vi "Initialize Array from Array.vi"   [LabVIEW 2009]
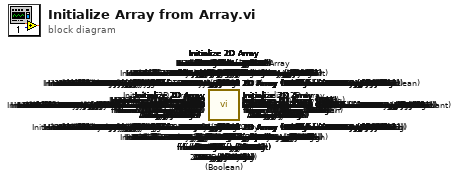
[diagram p0: block diagram]
diagram:
  n1 = call "Initialize 2D Array (Variant) from 2D Array (Variant).vi"() -> ()  [unwired: 2 in, 1 out]
  n2 = call "Initialize 2D Array (Variant) from 2D Array (U8).vi"() -> ()  [unwired: 2 in, 1 out]
  n3 = call "Initialize 2D Array (Variant) from 2D Array (U64) .vi"() -> ()  [unwired: 2 in, 1 out]
  n4 = call "Initialize 2D Array (Variant) from 2D Array (U32).vi"() -> ()  [unwired: 2 in, 1 out]
  n5 = call "Initialize 2D Array (Variant) from 2D Array (U16).vi"() -> ()  [unwired: 2 in, 1 out]
  n6 = call "Initialize 2D Array (Variant) from 2D Array (String).vi"() -> ()  [unwired: 2 in, 1 out]
  n7 = call "Initialize 2D Array (Variant) from 2D Array (SGL).vi"() -> ()  [unwired: 2 in, 1 out]
  n8 = call "Initialize 2D Array (Variant) from 2D Array (Path).vi"() -> ()  [unwired: 2 in, 1 out]
  n9 = call "Initialize 2D Array (Variant) from 2D Array (I8).vi"() -> ()  [unwired: 2 in, 1 out]
  n10 = call "Initialize 2D Array (Variant) from 2D Array (I64).vi"() -> ()  [unwired: 2 in, 1 out]
  n11 = call "Initialize 2D Array (Variant) from 2D Array (I32).vi"() -> ()  [unwired: 2 in, 1 out]
  n12 = call "Initialize 2D Array (Variant) from 2D Array (I16).vi"() -> ()  [unwired: 2 in, 1 out]
  n13 = call "Initialize 2D Array (Variant) from 2D Array (EXT).vi"() -> ()  [unwired: 2 in, 1 out]
  n14 = call "Initialize 2D Array (Variant) from 2D Array (DBL).vi"() -> ()  [unwired: 2 in, 1 out]
  n15 = call "Initialize 2D Array (Variant) from 2D Array (CXT).vi"() -> ()  [unwired: 2 in, 1 out]
  n16 = call "Initialize 2D Array (Variant) from 2D Array (CSG).vi"() -> ()  [unwired: 2 in, 1 out]
  n17 = call "Initialize 2D Array (Variant) from 2D Array (CDB).vi"() -> ()  [unwired: 2 in, 1 out]
  n18 = call "Initialize 2D Array (Variant) from 2D Array (Boolean).vi"() -> ()  [unwired: 2 in, 1 out]
  n19 = call "Initialize 2D Array (U8) from 2D Array (Variant).vi"() -> ()  [unwired: 2 in, 1 out]
  n20 = call "Initialize 2D Array (U8) from 2D Array (U8).vi"() -> ()  [unwired: 2 in, 1 out]
  n21 = call "Initialize 2D Array (U8) from 2D Array (U64) .vi"() -> ()  [unwired: 2 in, 1 out]
  n22 = call "Initialize 2D Array (U8) from 2D Array (U32).vi"() -> ()  [unwired: 2 in, 1 out]
  n23 = call "Initialize 2D Array (U8) from 2D Array (U16).vi"() -> ()  [unwired: 2 in, 1 out]
  n24 = call "Initialize 2D Array (U8) from 2D Array (String).vi"() -> ()  [unwired: 2 in, 1 out]
  n25 = call "Initialize 2D Array (U8) from 2D Array (SGL).vi"() -> ()  [unwired: 2 in, 1 out]
  n26 = call "Initialize 2D Array (U8) from 2D Array (Path).vi"() -> ()  [unwired: 2 in, 1 out]
  n27 = call "Initialize 2D Array (U8) from 2D Array (I8).vi"() -> ()  [unwired: 2 in, 1 out]
  n28 = call "Initialize 2D Array (U8) from 2D Array (I64).vi"() -> ()  [unwired: 2 in, 1 out]
  n29 = call "Initialize 2D Array (U8) from 2D Array (I32).vi"() -> ()  [unwired: 2 in, 1 out]
  n30 = call "Initialize 2D Array (U8) from 2D Array (I16).vi"() -> ()  [unwired: 2 in, 1 out]
  n31 = call "Initialize 2D Array (U8) from 2D Array (EXT).vi"() -> ()  [unwired: 2 in, 1 out]
  n32 = call "Initialize 2D Array (U8) from 2D Array (DBL).vi"() -> ()  [unwired: 2 in, 1 out]
  n33 = call "Initialize 2D Array (U8) from 2D Array (CXT).vi"() -> ()  [unwired: 2 in, 1 out]
  n34 = call "Initialize 2D Array (U8) from 2D Array (CSG).vi"() -> ()  [unwired: 2 in, 1 out]
  n35 = call "Initialize 2D Array (U8) from 2D Array (CDB).vi"() -> ()  [unwired: 2 in, 1 out]
  n36 = call "Initialize 2D Array (U8) from 2D Array (Boolean).vi"() -> ()  [unwired: 2 in, 1 out]
  n37 = call "Initialize 2D Array (U64) from 2D Array (Variant).vi"() -> ()  [unwired: 2 in, 1 out]
  n38 = call "Initialize 2D Array (U64) from 2D Array (U8).vi"() -> ()  [unwired: 2 in, 1 out]
  n39 = call "Initialize 2D Array (U64) from 2D Array (U64).vi"() -> ()  [unwired: 2 in, 1 out]
  n40 = call "Initialize 2D Array (U64) from 2D Array (U32).vi"() -> ()  [unwired: 2 in, 1 out]
  n41 = call "Initialize 2D Array (U64) from 2D Array (U16).vi"() -> ()  [unwired: 2 in, 1 out]
  n42 = call "Initialize 2D Array (U64) from 2D Array (String).vi"() -> ()  [unwired: 2 in, 1 out]
  n43 = call "Initialize 2D Array (U64) from 2D Array (SGL).vi"() -> ()  [unwired: 2 in, 1 out]
  n44 = call "Initialize 2D Array (U64) from 2D Array (Path).vi"() -> ()  [unwired: 2 in, 1 out]
  n45 = call "Initialize 2D Array (U64) from 2D Array (I8).vi"() -> ()  [unwired: 2 in, 1 out]
  n46 = call "Initialize 2D Array (U64) from 2D Array (I64).vi"() -> ()  [unwired: 2 in, 1 out]
  n47 = call "Initialize 2D Array (U64) from 2D Array (I32).vi"() -> ()  [unwired: 2 in, 1 out]
  n48 = call "Initialize 2D Array (U64) from 2D Array (I16).vi"() -> ()  [unwired: 2 in, 1 out]
  n49 = call "Initialize 2D Array (U64) from 2D Array (EXT).vi"() -> ()  [unwired: 2 in, 1 out]
  n50 = call "Initialize 2D Array (U64) from 2D Array (DBL).vi"() -> ()  [unwired: 2 in, 1 out]
  n51 = call "Initialize 2D Array (U64) from 2D Array (CXT).vi"() -> ()  [unwired: 2 in, 1 out]
  n52 = call "Initialize 2D Array (U64) from 2D Array (CSG).vi"() -> ()  [unwired: 2 in, 1 out]
  n53 = call "Initialize 2D Array (U64) from 2D Array (CDB).vi"() -> ()  [unwired: 2 in, 1 out]
  n54 = call "Initialize 2D Array (U64) from 2D Array (Boolean).vi"() -> ()  [unwired: 2 in, 1 out]
  n55 = call "Initialize 2D Array (U32) from 2D Array (Variant).vi"() -> ()  [unwired: 2 in, 1 out]
  n56 = call "Initialize 2D Array (U32) from 2D Array (U8).vi"() -> ()  [unwired: 2 in, 1 out]
  n57 = call "Initialize 2D Array (U32) from 2D Array (U64) .vi"() -> ()  [unwired: 2 in, 1 out]
  n58 = call "Initialize 2D Array (U32) from 2D Array (U32).vi"() -> ()  [unwired: 2 in, 1 out]
  n59 = call "Initialize 2D Array (U32) from 2D Array (U16).vi"() -> ()  [unwired: 2 in, 1 out]
  n60 = call "Initialize 2D Array (U32) from 2D Array (String).vi"() -> ()  [unwired: 2 in, 1 out]
  n61 = call "Initialize 2D Array (U32) from 2D Array (SGL).vi"() -> ()  [unwired: 2 in, 1 out]
  n62 = call "Initialize 2D Array (U32) from 2D Array (Path).vi"() -> ()  [unwired: 2 in, 1 out]
  n63 = call "Initialize 2D Array (U32) from 2D Array (I8).vi"() -> ()  [unwired: 2 in, 1 out]
  n64 = call "Initialize 2D Array (U32) from 2D Array (I64).vi"() -> ()  [unwired: 2 in, 1 out]
  n65 = call "Initialize 2D Array (U32) from 2D Array (I32).vi"() -> ()  [unwired: 2 in, 1 out]
  n66 = call "Initialize 2D Array (U32) from 2D Array (I16).vi"() -> ()  [unwired: 2 in, 1 out]
  n67 = call "Initialize 2D Array (U32) from 2D Array (EXT).vi"() -> ()  [unwired: 2 in, 1 out]
  n68 = call "Initialize 2D Array (U32) from 2D Array (DBL).vi"() -> ()  [unwired: 2 in, 1 out]
  n69 = call "Initialize 2D Array (U32) from 2D Array (CXT).vi"() -> ()  [unwired: 2 in, 1 out]
  n70 = call "Initialize 2D Array (U32) from 2D Array (CSG).vi"() -> ()  [unwired: 2 in, 1 out]
  n71 = call "Initialize 2D Array (U32) from 2D Array (CDB).vi"() -> ()  [unwired: 2 in, 1 out]
  n72 = call "Initialize 2D Array (U32) from 2D Array (Boolean).vi"() -> ()  [unwired: 2 in, 1 out]
  n73 = call "Initialize 2D Array (U16) from 2D Array (Variant).vi"() -> ()  [unwired: 2 in, 1 out]
  n74 = call "Initialize 2D Array (U16) from 2D Array (U8).vi"() -> ()  [unwired: 2 in, 1 out]
  n75 = call "Initialize 2D Array (U16) from 2D Array (U64) .vi"() -> ()  [unwired: 2 in, 1 out]
  n76 = call "Initialize 2D Array (U16) from 2D Array (U32).vi"() -> ()  [unwired: 2 in, 1 out]
  n77 = call "Initialize 2D Array (U16) from 2D Array (U16).vi"() -> ()  [unwired: 2 in, 1 out]
  n78 = call "Initialize 2D Array (U16) from 2D Array (String).vi"() -> ()  [unwired: 2 in, 1 out]
  n79 = call "Initialize 2D Array (U16) from 2D Array (SGL).vi"() -> ()  [unwired: 2 in, 1 out]
  n80 = call "Initialize 2D Array (U16) from 2D Array (Path).vi"() -> ()  [unwired: 2 in, 1 out]
  n81 = call "Initialize 2D Array (U16) from 2D Array (I8).vi"() -> ()  [unwired: 2 in, 1 out]
  n82 = call "Initialize 2D Array (U16) from 2D Array (I64).vi"() -> ()  [unwired: 2 in, 1 out]
  n83 = call "Initialize 2D Array (U16) from 2D Array (I32).vi"() -> ()  [unwired: 2 in, 1 out]
  n84 = call "Initialize 2D Array (U16) from 2D Array (I16).vi"() -> ()  [unwired: 2 in, 1 out]
  n85 = call "Initialize 2D Array (U16) from 2D Array (EXT).vi"() -> ()  [unwired: 2 in, 1 out]
  n86 = call "Initialize 2D Array (U16) from 2D Array (DBL).vi"() -> ()  [unwired: 2 in, 1 out]
  n87 = call "Initialize 2D Array (U16) from 2D Array (CXT).vi"() -> ()  [unwired: 2 in, 1 out]
  n88 = call "Initialize 2D Array (U16) from 2D Array (CSG).vi"() -> ()  [unwired: 2 in, 1 out]
  n89 = call "Initialize 2D Array (U16) from 2D Array (CDB).vi"() -> ()  [unwired: 2 in, 1 out]
  n90 = call "Initialize 2D Array (U16) from 2D Array (Boolean).vi"() -> ()  [unwired: 2 in, 1 out]
  n91 = call "Initialize 2D Array (String) from 2D Array (Variant).vi"() -> ()  [unwired: 2 in, 1 out]
  n92 = call "Initialize 2D Array (String) from 2D Array (U8).vi"() -> ()  [unwired: 2 in, 1 out]
  n93 = call "Initialize 2D Array (String) from 2D Array (U64) .vi"() -> ()  [unwired: 2 in, 1 out]
  n94 = call "Initialize 2D Array (String) from 2D Array (U32).vi"() -> ()  [unwired: 2 in, 1 out]
  n95 = call "Initialize 2D Array (String) from 2D Array (U16).vi"() -> ()  [unwired: 2 in, 1 out]
  n96 = call "Initialize 2D Array (String) from 2D Array (String).vi"() -> ()  [unwired: 2 in, 1 out]
  n97 = call "Initialize 2D Array (String) from 2D Array (SGL).vi"() -> ()  [unwired: 2 in, 1 out]
  n98 = call "Initialize 2D Array (String) from 2D Array (Path).vi"() -> ()  [unwired: 2 in, 1 out]
  n99 = call "Initialize 2D Array (String) from 2D Array (I8).vi"() -> ()  [unwired: 2 in, 1 out]
  n100 = call "Initialize 2D Array (String) from 2D Array (I64).vi"() -> ()  [unwired: 2 in, 1 out]
  n101 = call "Initialize 2D Array (String) from 2D Array (I32).vi"() -> ()  [unwired: 2 in, 1 out]
  n102 = call "Initialize 2D Array (String) from 2D Array (I16).vi"() -> ()  [unwired: 2 in, 1 out]
  n103 = call "Initialize 2D Array (String) from 2D Array (EXT).vi"() -> ()  [unwired: 2 in, 1 out]
  n104 = call "Initialize 2D Array (String) from 2D Array (DBL).vi"() -> ()  [unwired: 2 in, 1 out]
  n105 = call "Initialize 2D Array (String) from 2D Array (CXT).vi"() -> ()  [unwired: 2 in, 1 out]
  n106 = call "Initialize 2D Array (String) from 2D Array (CSG).vi"() -> ()  [unwired: 2 in, 1 out]
  n107 = call "Initialize 2D Array (String) from 2D Array (CDB).vi"() -> ()  [unwired: 2 in, 1 out]
  n108 = call "Initialize 2D Array (String) from 2D Array (Boolean).vi"() -> ()  [unwired: 2 in, 1 out]
  n109 = call "Initialize 2D Array (SGL) from 2D Array (Variant).vi"() -> ()  [unwired: 2 in, 1 out]
  n110 = call "Initialize 2D Array (SGL) from 2D Array (U8).vi"() -> ()  [unwired: 2 in, 1 out]
  n111 = call "Initialize 2D Array (SGL) from 2D Array (U64) .vi"() -> ()  [unwired: 2 in, 1 out]
  n112 = call "Initialize 2D Array (SGL) from 2D Array (U32).vi"() -> ()  [unwired: 2 in, 1 out]
  n113 = call "Initialize 2D Array (SGL) from 2D Array (U16).vi"() -> ()  [unwired: 2 in, 1 out]
  n114 = call "Initialize 2D Array (SGL) from 2D Array (String).vi"() -> ()  [unwired: 2 in, 1 out]
  n115 = call "Initialize 2D Array (SGL) from 2D Array (SGL).vi"() -> ()  [unwired: 2 in, 1 out]
  n116 = call "Initialize 2D Array (SGL) from 2D Array (Path).vi"() -> ()  [unwired: 2 in, 1 out]
  n117 = call "Initialize 2D Array (SGL) from 2D Array (I8).vi"() -> ()  [unwired: 2 in, 1 out]
  n118 = call "Initialize 2D Array (SGL) from 2D Array (I64).vi"() -> ()  [unwired: 2 in, 1 out]
  n119 = call "Initialize 2D Array (SGL) from 2D Array (I32).vi"() -> ()  [unwired: 2 in, 1 out]
  n120 = call "Initialize 2D Array (SGL) from 2D Array (I16).vi"() -> ()  [unwired: 2 in, 1 out]
  n121 = call "Initialize 2D Array (SGL) from 2D Array (EXT).vi"() -> ()  [unwired: 2 in, 1 out]
  n122 = call "Initialize 2D Array (SGL) from 2D Array (DBL).vi"() -> ()  [unwired: 2 in, 1 out]
  n123 = call "Initialize 2D Array (SGL) from 2D Array (CXT).vi"() -> ()  [unwired: 2 in, 1 out]
  n124 = call "Initialize 2D Array (SGL) from 2D Array (CSG).vi"() -> ()  [unwired: 2 in, 1 out]
  n125 = call "Initialize 2D Array (SGL) from 2D Array (CDB).vi"() -> ()  [unwired: 2 in, 1 out]
  n126 = call "Initialize 2D Array (SGL) from 2D Array (Boolean).vi"() -> ()  [unwired: 2 in, 1 out]
  n127 = call "Initialize 2D Array (Path) from 2D Array (Variant).vi"() -> ()  [unwired: 2 in, 1 out]
  n128 = call "Initialize 2D Array (Path) from 2D Array (U8).vi"() -> ()  [unwired: 2 in, 1 out]
  n129 = call "Initialize 2D Array (Path) from 2D Array (U64) .vi"() -> ()  [unwired: 2 in, 1 out]
  n130 = call "Initialize 2D Array (Path) from 2D Array (U32).vi"() -> ()  [unwired: 2 in, 1 out]
  n131 = call "Initialize 2D Array (Path) from 2D Array (U16).vi"() -> ()  [unwired: 2 in, 1 out]
  n132 = call "Initialize 2D Array (Path) from 2D Array (String).vi"() -> ()  [unwired: 2 in, 1 out]
  n133 = call "Initialize 2D Array (Path) from 2D Array (SGL).vi"() -> ()  [unwired: 2 in, 1 out]
  n134 = call "Initialize 2D Array (Path) from 2D Array (Path).vi"() -> ()  [unwired: 2 in, 1 out]
  n135 = call "Initialize 2D Array (Path) from 2D Array (I8).vi"() -> ()  [unwired: 2 in, 1 out]
  n136 = call "Initialize 2D Array (Path) from 2D Array (I64).vi"() -> ()  [unwired: 2 in, 1 out]
  n137 = call "Initialize 2D Array (Path) from 2D Array (I32).vi"() -> ()  [unwired: 2 in, 1 out]
  n138 = call "Initialize 2D Array (Path) from 2D Array (I16).vi"() -> ()  [unwired: 2 in, 1 out]
  n139 = call "Initialize 2D Array (Path) from 2D Array (EXT).vi"() -> ()  [unwired: 2 in, 1 out]
  n140 = call "Initialize 2D Array (Path) from 2D Array (DBL).vi"() -> ()  [unwired: 2 in, 1 out]
  n141 = call "Initialize 2D Array (Path) from 2D Array (CXT).vi"() -> ()  [unwired: 2 in, 1 out]
  n142 = call "Initialize 2D Array (Path) from 2D Array (CSG).vi"() -> ()  [unwired: 2 in, 1 out]
  n143 = call "Initialize 2D Array (Path) from 2D Array (CDB).vi"() -> ()  [unwired: 2 in, 1 out]
  n144 = call "Initialize 2D Array (Path) from 2D Array (Boolean).vi"() -> ()  [unwired: 2 in, 1 out]
  n145 = call "Initialize 2D Array (I8) from 2D Array (Variant).vi"() -> ()  [unwired: 2 in, 1 out]
  n146 = call "Initialize 2D Array (I8) from 2D Array (U8).vi"() -> ()  [unwired: 2 in, 1 out]
  n147 = call "Initialize 2D Array (I8) from 2D Array (U64) .vi"() -> ()  [unwired: 2 in, 1 out]
  n148 = call "Initialize 2D Array (I8) from 2D Array (U32).vi"() -> ()  [unwired: 2 in, 1 out]
  n149 = call "Initialize 2D Array (I8) from 2D Array (U16).vi"() -> ()  [unwired: 2 in, 1 out]
  n150 = call "Initialize 2D Array (I8) from 2D Array (String).vi"() -> ()  [unwired: 2 in, 1 out]
  n151 = call "Initialize 2D Array (I8) from 2D Array (SGL).vi"() -> ()  [unwired: 2 in, 1 out]
  n152 = call "Initialize 2D Array (I8) from 2D Array (Path).vi"() -> ()  [unwired: 2 in, 1 out]
  n153 = call "Initialize 2D Array (I8) from 2D Array (I8).vi"() -> ()  [unwired: 2 in, 1 out]
  n154 = call "Initialize 2D Array (I8) from 2D Array (I64).vi"() -> ()  [unwired: 2 in, 1 out]
  n155 = call "Initialize 2D Array (I8) from 2D Array (I32).vi"() -> ()  [unwired: 2 in, 1 out]
  n156 = call "Initialize 2D Array (I8) from 2D Array (I16).vi"() -> ()  [unwired: 2 in, 1 out]
  n157 = call "Initialize 2D Array (I8) from 2D Array (EXT).vi"() -> ()  [unwired: 2 in, 1 out]
  n158 = call "Initialize 2D Array (I8) from 2D Array (DBL).vi"() -> ()  [unwired: 2 in, 1 out]
  n159 = call "Initialize 2D Array (I8) from 2D Array (CXT).vi"() -> ()  [unwired: 2 in, 1 out]
  n160 = call "Initialize 2D Array (I8) from 2D Array (CSG).vi"() -> ()  [unwired: 2 in, 1 out]
  n161 = call "Initialize 2D Array (I8) from 2D Array (CDB).vi"() -> ()  [unwired: 2 in, 1 out]
  n162 = call "Initialize 2D Array (I8) from 2D Array (Boolean).vi"() -> ()  [unwired: 2 in, 1 out]
  n163 = call "Initialize 2D Array (I64) from 2D Array (Variant).vi"() -> ()  [unwired: 2 in, 1 out]
  n164 = call "Initialize 2D Array (I64) from 2D Array (U8).vi"() -> ()  [unwired: 2 in, 1 out]
  n165 = call "Initialize 2D Array (I64) from 2D Array (U64).vi"() -> ()  [unwired: 2 in, 1 out]
  n166 = call "Initialize 2D Array (I64) from 2D Array (U32).vi"() -> ()  [unwired: 2 in, 1 out]
  n167 = call "Initialize 2D Array (I64) from 2D Array (U16).vi"() -> ()  [unwired: 2 in, 1 out]
  n168 = call "Initialize 2D Array (I64) from 2D Array (String).vi"() -> ()  [unwired: 2 in, 1 out]
  n169 = call "Initialize 2D Array (I64) from 2D Array (SGL).vi"() -> ()  [unwired: 2 in, 1 out]
  n170 = call "Initialize 2D Array (I64) from 2D Array (Path).vi"() -> ()  [unwired: 2 in, 1 out]
  n171 = call "Initialize 2D Array (I64) from 2D Array (I8).vi"() -> ()  [unwired: 2 in, 1 out]
  n172 = call "Initialize 2D Array (I64) from 2D Array (I64).vi"() -> ()  [unwired: 2 in, 1 out]
  n173 = call "Initialize 2D Array (I64) from 2D Array (I32).vi"() -> ()  [unwired: 2 in, 1 out]
  n174 = call "Initialize 2D Array (I64) from 2D Array (I16).vi"() -> ()  [unwired: 2 in, 1 out]
  n175 = call "Initialize 2D Array (I64) from 2D Array (EXT).vi"() -> ()  [unwired: 2 in, 1 out]
  n176 = call "Initialize 2D Array (I64) from 2D Array (DBL).vi"() -> ()  [unwired: 2 in, 1 out]
  n177 = call "Initialize 2D Array (I64) from 2D Array (CXT).vi"() -> ()  [unwired: 2 in, 1 out]
  n178 = call "Initialize 2D Array (I64) from 2D Array (CSG).vi"() -> ()  [unwired: 2 in, 1 out]
  n179 = call "Initialize 2D Array (I64) from 2D Array (CDB).vi"() -> ()  [unwired: 2 in, 1 out]
  n180 = call "Initialize 2D Array (I64) from 2D Array (Boolean).vi"() -> ()  [unwired: 2 in, 1 out]
  n181 = call "Initialize 2D Array (I32) from 2D Array (Variant).vi"() -> ()  [unwired: 2 in, 1 out]
  n182 = call "Initialize 2D Array (I32) from 2D Array (U8).vi"() -> ()  [unwired: 2 in, 1 out]
  n183 = call "Initialize 2D Array (I32) from 2D Array (U64) .vi"() -> ()  [unwired: 2 in, 1 out]
  n184 = call "Initialize 2D Array (I32) from 2D Array (U32).vi"() -> ()  [unwired: 2 in, 1 out]
  n185 = call "Initialize 2D Array (I32) from 2D Array (U16).vi"() -> ()  [unwired: 2 in, 1 out]
  n186 = call "Initialize 2D Array (I32) from 2D Array (String).vi"() -> ()  [unwired: 2 in, 1 out]
  n187 = call "Initialize 2D Array (I32) from 2D Array (SGL).vi"() -> ()  [unwired: 2 in, 1 out]
  n188 = call "Initialize 2D Array (I32) from 2D Array (Path).vi"() -> ()  [unwired: 2 in, 1 out]
  n189 = call "Initialize 2D Array (I32) from 2D Array (I8).vi"() -> ()  [unwired: 2 in, 1 out]
  n190 = call "Initialize 2D Array (I32) from 2D Array (I64).vi"() -> ()  [unwired: 2 in, 1 out]
  n191 = call "Initialize 2D Array (I32) from 2D Array (I32).vi"() -> ()  [unwired: 2 in, 1 out]
  n192 = call "Initialize 2D Array (I32) from 2D Array (I16).vi"() -> ()  [unwired: 2 in, 1 out]
  n193 = call "Initialize 2D Array (I32) from 2D Array (EXT).vi"() -> ()  [unwired: 2 in, 1 out]
  n194 = call "Initialize 2D Array (I32) from 2D Array (DBL).vi"() -> ()  [unwired: 2 in, 1 out]
  n195 = call "Initialize 2D Array (I32) from 2D Array (CXT).vi"() -> ()  [unwired: 2 in, 1 out]
  n196 = call "Initialize 2D Array (I32) from 2D Array (CSG).vi"() -> ()  [unwired: 2 in, 1 out]
  n197 = call "Initialize 2D Array (I32) from 2D Array (CDB).vi"() -> ()  [unwired: 2 in, 1 out]
  n198 = call "Initialize 2D Array (I32) from 2D Array (Boolean).vi"() -> ()  [unwired: 2 in, 1 out]
  n199 = call "Initialize 2D Array (I16) from 2D Array (Variant).vi"() -> ()  [unwired: 2 in, 1 out]
  n200 = call "Initialize 2D Array (I16) from 2D Array (U8).vi"() -> ()  [unwired: 2 in, 1 out]
  n201 = call "Initialize 2D Array (I16) from 2D Array (U64) .vi"() -> ()  [unwired: 2 in, 1 out]
  n202 = call "Initialize 2D Array (I16) from 2D Array (U32).vi"() -> ()  [unwired: 2 in, 1 out]
  n203 = call "Initialize 2D Array (I16) from 2D Array (U16).vi"() -> ()  [unwired: 2 in, 1 out]
  n204 = call "Initialize 2D Array (I16) from 2D Array (String).vi"() -> ()  [unwired: 2 in, 1 out]
  n205 = call "Initialize 2D Array (I16) from 2D Array (SGL).vi"() -> ()  [unwired: 2 in, 1 out]
  n206 = call "Initialize 2D Array (I16) from 2D Array (Path).vi"() -> ()  [unwired: 2 in, 1 out]
  n207 = call "Initialize 2D Array (I16) from 2D Array (I8).vi"() -> ()  [unwired: 2 in, 1 out]
  n208 = call "Initialize 2D Array (I16) from 2D Array (I64).vi"() -> ()  [unwired: 2 in, 1 out]
  n209 = call "Initialize 2D Array (I16) from 2D Array (I32).vi"() -> ()  [unwired: 2 in, 1 out]
  n210 = call "Initialize 2D Array (I16) from 2D Array (I16).vi"() -> ()  [unwired: 2 in, 1 out]
  n211 = call "Initialize 2D Array (I16) from 2D Array (EXT).vi"() -> ()  [unwired: 2 in, 1 out]
  n212 = call "Initialize 2D Array (I16) from 2D Array (DBL).vi"() -> ()  [unwired: 2 in, 1 out]
  n213 = call "Initialize 2D Array (I16) from 2D Array (CXT).vi"() -> ()  [unwired: 2 in, 1 out]
  n214 = call "Initialize 2D Array (I16) from 2D Array (CSG).vi"() -> ()  [unwired: 2 in, 1 out]
  n215 = call "Initialize 2D Array (I16) from 2D Array (CDB).vi"() -> ()  [unwired: 2 in, 1 out]
  n216 = call "Initialize 2D Array (I16) from 2D Array (Boolean).vi"() -> ()  [unwired: 2 in, 1 out]
  n217 = call "Initialize 2D Array (EXT) from 2D Array (Variant).vi"() -> ()  [unwired: 2 in, 1 out]
  n218 = call "Initialize 2D Array (EXT) from 2D Array (U8).vi"() -> ()  [unwired: 2 in, 1 out]
  n219 = call "Initialize 2D Array (EXT) from 2D Array (U64) .vi"() -> ()  [unwired: 2 in, 1 out]
  n220 = call "Initialize 2D Array (EXT) from 2D Array (U32).vi"() -> ()  [unwired: 2 in, 1 out]
  n221 = call "Initialize 2D Array (EXT) from 2D Array (U16).vi"() -> ()  [unwired: 2 in, 1 out]
  n222 = call "Initialize 2D Array (EXT) from 2D Array (String).vi"() -> ()  [unwired: 2 in, 1 out]
  n223 = call "Initialize 2D Array (EXT) from 2D Array (SGL).vi"() -> ()  [unwired: 2 in, 1 out]
  n224 = call "Initialize 2D Array (EXT) from 2D Array (Path).vi"() -> ()  [unwired: 2 in, 1 out]
  n225 = call "Initialize 2D Array (EXT) from 2D Array (I8).vi"() -> ()  [unwired: 2 in, 1 out]
  n226 = call "Initialize 2D Array (EXT) from 2D Array (I64).vi"() -> ()  [unwired: 2 in, 1 out]
  n227 = call "Initialize 2D Array (EXT) from 2D Array (I32).vi"() -> ()  [unwired: 2 in, 1 out]
  n228 = call "Initialize 2D Array (EXT) from 2D Array (I16).vi"() -> ()  [unwired: 2 in, 1 out]
  n229 = call "Initialize 2D Array (EXT) from 2D Array (EXT).vi"() -> ()  [unwired: 2 in, 1 out]
  n230 = call "Initialize 2D Array (EXT) from 2D Array (DBL).vi"() -> ()  [unwired: 2 in, 1 out]
  n231 = call "Initialize 2D Array (EXT) from 2D Array (CXT).vi"() -> ()  [unwired: 2 in, 1 out]
  n232 = call "Initialize 2D Array (EXT) from 2D Array (CSG).vi"() -> ()  [unwired: 2 in, 1 out]
  n233 = call "Initialize 2D Array (EXT) from 2D Array (CDB).vi"() -> ()  [unwired: 2 in, 1 out]
  n234 = call "Initialize 2D Array (EXT) from 2D Array (Boolean).vi"() -> ()  [unwired: 2 in, 1 out]
  n235 = call "Initialize 2D Array (DBL) from 2D Array (Variant).vi"() -> ()  [unwired: 2 in, 1 out]
  n236 = call "Initialize 2D Array (DBL) from 2D Array (U8).vi"() -> ()  [unwired: 2 in, 1 out]
  n237 = call "Initialize 2D Array (DBL) from 2D Array (U64) .vi"() -> ()  [unwired: 2 in, 1 out]
  n238 = call "Initialize 2D Array (DBL) from 2D Array (U32).vi"() -> ()  [unwired: 2 in, 1 out]
  n239 = call "Initialize 2D Array (DBL) from 2D Array (U16).vi"() -> ()  [unwired: 2 in, 1 out]
  n240 = call "Initialize 2D Array (DBL) from 2D Array (String).vi"() -> ()  [unwired: 2 in, 1 out]
  n241 = call "Initialize 2D Array (DBL) from 2D Array (SGL).vi"() -> ()  [unwired: 2 in, 1 out]
  n242 = call "Initialize 2D Array (DBL) from 2D Array (Path).vi"() -> ()  [unwired: 2 in, 1 out]
  n243 = call "Initialize 2D Array (DBL) from 2D Array (I8).vi"() -> ()  [unwired: 2 in, 1 out]
  n244 = call "Initialize 2D Array (DBL) from 2D Array (I64).vi"() -> ()  [unwired: 2 in, 1 out]
  n245 = call "Initialize 2D Array (DBL) from 2D Array (I32).vi"() -> ()  [unwired: 2 in, 1 out]
  n246 = call "Initialize 2D Array (DBL) from 2D Array (I16).vi"() -> ()  [unwired: 2 in, 1 out]
  n247 = call "Initialize 2D Array (DBL) from 2D Array (EXT).vi"() -> ()  [unwired: 2 in, 1 out]
  n248 = call "Initialize 2D Array (DBL) from 2D Array (DBL).vi"() -> ()  [unwired: 2 in, 1 out]
  n249 = call "Initialize 2D Array (DBL) from 2D Array (CXT).vi"() -> ()  [unwired: 2 in, 1 out]
  n250 = call "Initialize 2D Array (DBL) from 2D Array (CSG).vi"() -> ()  [unwired: 2 in, 1 out]
  n251 = call "Initialize 2D Array (DBL) from 2D Array (CDB).vi"() -> ()  [unwired: 2 in, 1 out]
  n252 = call "Initialize 2D Array (DBL) from 2D Array (Boolean).vi"() -> ()  [unwired: 2 in, 1 out]
  n253 = call "Initialize 2D Array (CXT) from 2D Array (Variant).vi"() -> ()  [unwired: 2 in, 1 out]
  n254 = call "Initialize 2D Array (CXT) from 2D Array (U8).vi"() -> ()  [unwired: 2 in, 1 out]
  n255 = call "Initialize 2D Array (CXT) from 2D Array (U64) .vi"() -> ()  [unwired: 2 in, 1 out]
  n256 = call "Initialize 2D Array (CXT) from 2D Array (U32).vi"() -> ()  [unwired: 2 in, 1 out]
  n257 = call "Initialize 2D Array (CXT) from 2D Array (U16).vi"() -> ()  [unwired: 2 in, 1 out]
  n258 = call "Initialize 2D Array (CXT) from 2D Array (String).vi"() -> ()  [unwired: 2 in, 1 out]
  n259 = call "Initialize 2D Array (CXT) from 2D Array (SGL).vi"() -> ()  [unwired: 2 in, 1 out]
  n260 = call "Initialize 2D Array (CXT) from 2D Array (Path).vi"() -> ()  [unwired: 2 in, 1 out]
  n261 = call "Initialize 2D Array (CXT) from 2D Array (I8).vi"() -> ()  [unwired: 2 in, 1 out]
  n262 = call "Initialize 2D Array (CXT) from 2D Array (I64).vi"() -> ()  [unwired: 2 in, 1 out]
  n263 = call "Initialize 2D Array (CXT) from 2D Array (I32).vi"() -> ()  [unwired: 2 in, 1 out]
  n264 = call "Initialize 2D Array (CXT) from 2D Array (I16).vi"() -> ()  [unwired: 2 in, 1 out]
  n265 = call "Initialize 2D Array (CXT) from 2D Array (EXT).vi"() -> ()  [unwired: 2 in, 1 out]
  n266 = call "Initialize 2D Array (CXT) from 2D Array (DBL).vi"() -> ()  [unwired: 2 in, 1 out]
  n267 = call "Initialize 2D Array (CXT) from 2D Array (CXT).vi"() -> ()  [unwired: 2 in, 1 out]
  n268 = call "Initialize 2D Array (CXT) from 2D Array (CSG).vi"() -> ()  [unwired: 2 in, 1 out]
  n269 = call "Initialize 2D Array (CXT) from 2D Array (CDB).vi"() -> ()  [unwired: 2 in, 1 out]
  n270 = call "Initialize 2D Array (CXT) from 2D Array (Boolean).vi"() -> ()  [unwired: 2 in, 1 out]
  n271 = call "Initialize 2D Array (CSG) from 2D Array (Variant).vi"() -> ()  [unwired: 2 in, 1 out]
  n272 = call "Initialize 2D Array (CSG) from 2D Array (U8).vi"() -> ()  [unwired: 2 in, 1 out]
  n273 = call "Initialize 2D Array (CSG) from 2D Array (U64) .vi"() -> ()  [unwired: 2 in, 1 out]
  n274 = call "Initialize 2D Array (CSG) from 2D Array (U32).vi"() -> ()  [unwired: 2 in, 1 out]
  n275 = call "Initialize 2D Array (CSG) from 2D Array (U16).vi"() -> ()  [unwired: 2 in, 1 out]
  n276 = call "Initialize 2D Array (CSG) from 2D Array (String).vi"() -> ()  [unwired: 2 in, 1 out]
  n277 = call "Initialize 2D Array (CSG) from 2D Array (SGL).vi"() -> ()  [unwired: 2 in, 1 out]
  n278 = call "Initialize 2D Array (CSG) from 2D Array (Path).vi"() -> ()  [unwired: 2 in, 1 out]
  n279 = call "Initialize 2D Array (CSG) from 2D Array (I8).vi"() -> ()  [unwired: 2 in, 1 out]
  n280 = call "Initialize 2D Array (CSG) from 2D Array (I64).vi"() -> ()  [unwired: 2 in, 1 out]
  n281 = call "Initialize 2D Array (CSG) from 2D Array (I32).vi"() -> ()  [unwired: 2 in, 1 out]
  n282 = call "Initialize 2D Array (CSG) from 2D Array (I16).vi"() -> ()  [unwired: 2 in, 1 out]
  n283 = call "Initialize 2D Array (CSG) from 2D Array (EXT).vi"() -> ()  [unwired: 2 in, 1 out]
  n284 = call "Initialize 2D Array (CSG) from 2D Array (DBL).vi"() -> ()  [unwired: 2 in, 1 out]
  n285 = call "Initialize 2D Array (CSG) from 2D Array (CXT).vi"() -> ()  [unwired: 2 in, 1 out]
  n286 = call "Initialize 2D Array (CSG) from 2D Array (CSG).vi"() -> ()  [unwired: 2 in, 1 out]
  n287 = call "Initialize 2D Array (CSG) from 2D Array (CDB).vi"() -> ()  [unwired: 2 in, 1 out]
  n288 = call "Initialize 2D Array (CSG) from 2D Array (Boolean).vi"() -> ()  [unwired: 2 in, 1 out]
  n289 = call "Initialize 2D Array (CDB) from 2D Array (Variant).vi"() -> ()  [unwired: 2 in, 1 out]
  n290 = call "Initialize 2D Array (CDB) from 2D Array (U8).vi"() -> ()  [unwired: 2 in, 1 out]
  n291 = call "Initialize 2D Array (CDB) from 2D Array (U64) .vi"() -> ()  [unwired: 2 in, 1 out]
  n292 = call "Initialize 2D Array (CDB) from 2D Array (U32).vi"() -> ()  [unwired: 2 in, 1 out]
  n293 = call "Initialize 2D Array (CDB) from 2D Array (U16).vi"() -> ()  [unwired: 2 in, 1 out]
  n294 = call "Initialize 2D Array (CDB) from 2D Array (String).vi"() -> ()  [unwired: 2 in, 1 out]
  n295 = call "Initialize 2D Array (CDB) from 2D Array (SGL).vi"() -> ()  [unwired: 2 in, 1 out]
  n296 = call "Initialize 2D Array (CDB) from 2D Array (Path).vi"() -> ()  [unwired: 2 in, 1 out]
  n297 = call "Initialize 2D Array (CDB) from 2D Array (I8).vi"() -> ()  [unwired: 2 in, 1 out]
  n298 = call "Initialize 2D Array (CDB) from 2D Array (I64).vi"() -> ()  [unwired: 2 in, 1 out]
  n299 = call "Initialize 2D Array (CDB) from 2D Array (I32).vi"() -> ()  [unwired: 2 in, 1 out]
  n300 = call "Initialize 2D Array (CDB) from 2D Array (I16).vi"() -> ()  [unwired: 2 in, 1 out]
  n301 = call "Initialize 2D Array (CDB) from 2D Array (EXT).vi"() -> ()  [unwired: 2 in, 1 out]
  n302 = call "Initialize 2D Array (CDB) from 2D Array (DBL).vi"() -> ()  [unwired: 2 in, 1 out]
  n303 = call "Initialize 2D Array (CDB) from 2D Array (CXT).vi"() -> ()  [unwired: 2 in, 1 out]
  n304 = call "Initialize 2D Array (CDB) from 2D Array (CSG).vi"() -> ()  [unwired: 2 in, 1 out]
  n305 = call "Initialize 2D Array (CDB) from 2D Array (CDB).vi"() -> ()  [unwired: 2 in, 1 out]
  n306 = call "Initialize 2D Array (CDB) from 2D Array (Boolean).vi"() -> ()  [unwired: 2 in, 1 out]
  n307 = call "Initialize 2D Array (Boolean) from 2D Array (Variant).vi"() -> ()  [unwired: 2 in, 1 out]
  n308 = call "Initialize 2D Array (Boolean) from 2D Array (U8).vi"() -> ()  [unwired: 2 in, 1 out]
  n309 = call "Initialize 2D Array (Boolean) from 2D Array (U64) .vi"() -> ()  [unwired: 2 in, 1 out]
  n310 = call "Initialize 2D Array (Boolean) from 2D Array (U32).vi"() -> ()  [unwired: 2 in, 1 out]
  n311 = call "Initialize 2D Array (Boolean) from 2D Array (U16).vi"() -> ()  [unwired: 2 in, 1 out]
  n312 = call "Initialize 2D Array (Boolean) from 2D Array (String).vi"() -> ()  [unwired: 2 in, 1 out]
  n313 = call "Initialize 2D Array (Boolean) from 2D Array (SGL).vi"() -> ()  [unwired: 2 in, 1 out]
  n314 = call "Initialize 2D Array (Boolean) from 2D Array (Path).vi"() -> ()  [unwired: 2 in, 1 out]
  n315 = call "Initialize 2D Array (Boolean) from 2D Array (I8).vi"() -> ()  [unwired: 2 in, 1 out]
  n316 = call "Initialize 2D Array (Boolean) from 2D Array (I64).vi"() -> ()  [unwired: 2 in, 1 out]
  n317 = call "Initialize 2D Array (Boolean) from 2D Array (I32).vi"() -> ()  [unwired: 2 in, 1 out]
  n318 = call "Initialize 2D Array (Boolean) from 2D Array (I16).vi"() -> ()  [unwired: 2 in, 1 out]
  n319 = call "Initialize 2D Array (Boolean) from 2D Array (EXT).vi"() -> ()  [unwired: 2 in, 1 out]
  n320 = call "Initialize 2D Array (Boolean) from 2D Array (DBL).vi"() -> ()  [unwired: 2 in, 1 out]
  n321 = call "Initialize 2D Array (Boolean) from 2D Array (CXT).vi"() -> ()  [unwired: 2 in, 1 out]
  n322 = call "Initialize 2D Array (Boolean) from 2D Array (CSG).vi"() -> ()  [unwired: 2 in, 1 out]
  n323 = call "Initialize 2D Array (Boolean) from 2D Array (CDB).vi"() -> ()  [unwired: 2 in, 1 out]
  n324 = call "Initialize 2D Array (Boolean) from 2D Array (Boolean).vi"() -> ()  [unwired: 2 in, 1 out]
  n325 = call "Initialize 1D Array (Variant) from 1D Array (Variant).vi"() -> ()  [unwired: 2 in, 1 out]
  n326 = call "Initialize 1D Array (Variant) from 1D Array (U8).vi"() -> ()  [unwired: 2 in, 1 out]
  n327 = call "Initialize 1D Array (Variant) from 1D Array (U64).vi"() -> ()  [unwired: 2 in, 1 out]
  n328 = call "Initialize 1D Array (Variant) from 1D Array (U32).vi"() -> ()  [unwired: 2 in, 1 out]
  n329 = call "Initialize 1D Array (Variant) from 1D Array (U16).vi"() -> ()  [unwired: 2 in, 1 out]
  n330 = call "Initialize 1D Array (Variant) from 1D Array (String).vi"() -> ()  [unwired: 2 in, 1 out]
  n331 = call "Initialize 1D Array (Variant) from 1D Array (SGL).vi"() -> ()  [unwired: 2 in, 1 out]
  n332 = call "Initialize 1D Array (Variant) from 1D Array (Path).vi"() -> ()  [unwired: 2 in, 1 out]
  n333 = call "Initialize 1D Array (Variant) from 1D Array (I8).vi"() -> ()  [unwired: 2 in, 1 out]
  n334 = call "Initialize 1D Array (Variant) from 1D Array (I64).vi"() -> ()  [unwired: 2 in, 1 out]
  n335 = call "Initialize 1D Array (Variant) from 1D Array (I32).vi"() -> ()  [unwired: 2 in, 1 out]
  n336 = call "Initialize 1D Array (Variant) from 1D Array (I16).vi"() -> ()  [unwired: 2 in, 1 out]
  n337 = call "Initialize 1D Array (Variant) from 1D Array (EXT).vi"() -> ()  [unwired: 2 in, 1 out]
  n338 = call "Initialize 1D Array (Variant) from 1D Array (DBL).vi"() -> ()  [unwired: 2 in, 1 out]
  n339 = call "Initialize 1D Array (Variant) from 1D Array (CXT).vi"() -> ()  [unwired: 2 in, 1 out]
  n340 = call "Initialize 1D Array (Variant) from 1D Array (CSG).vi"() -> ()  [unwired: 2 in, 1 out]
  n341 = call "Initialize 1D Array (Variant) from 1D Array (CDB).vi"() -> ()  [unwired: 2 in, 1 out]
  n342 = call "Initialize 1D Array (Variant) from 1D Array (Boolean).vi"() -> ()  [unwired: 2 in, 1 out]
  n343 = call "Initialize 1D Array (U8) from 1D Array (Variant).vi"() -> ()  [unwired: 2 in, 1 out]
  n344 = call "Initialize 1D Array (U8) from 1D Array (U8).vi"() -> ()  [unwired: 2 in, 1 out]
  n345 = call "Initialize 1D Array (U8) from 1D Array (U64).vi"() -> ()  [unwired: 2 in, 1 out]
  n346 = call "Initialize 1D Array (U8) from 1D Array (U32).vi"() -> ()  [unwired: 2 in, 1 out]
  n347 = call "Initialize 1D Array (U8) from 1D Array (U16).vi"() -> ()  [unwired: 2 in, 1 out]
  n348 = call "Initialize 1D Array (U8) from 1D Array (String).vi"() -> ()  [unwired: 2 in, 1 out]
  n349 = call "Initialize 1D Array (U8) from 1D Array (SGL).vi"() -> ()  [unwired: 2 in, 1 out]
  n350 = call "Initialize 1D Array (U8) from 1D Array (Path).vi"() -> ()  [unwired: 2 in, 1 out]
  n351 = call "Initialize 1D Array (U8) from 1D Array (I8).vi"() -> ()  [unwired: 2 in, 1 out]
  n352 = call "Initialize 1D Array (U8) from 1D Array (I64).vi"() -> ()  [unwired: 2 in, 1 out]
  n353 = call "Initialize 1D Array (U8) from 1D Array (I32).vi"() -> ()  [unwired: 2 in, 1 out]
  n354 = call "Initialize 1D Array (U8) from 1D Array (I16).vi"() -> ()  [unwired: 2 in, 1 out]
  n355 = call "Initialize 1D Array (U8) from 1D Array (EXT).vi"() -> ()  [unwired: 2 in, 1 out]
  n356 = call "Initialize 1D Array (U8) from 1D Array (DBL).vi"() -> ()  [unwired: 2 in, 1 out]
  n357 = call "Initialize 1D Array (U8) from 1D Array (CXT).vi"() -> ()  [unwired: 2 in, 1 out]
  n358 = call "Initialize 1D Array (U8) from 1D Array (CSG).vi"() -> ()  [unwired: 2 in, 1 out]
  n359 = call "Initialize 1D Array (U8) from 1D Array (CDB).vi"() -> ()  [unwired: 2 in, 1 out]
  n360 = call "Initialize 1D Array (U8) from 1D Array (Boolean).vi"() -> ()  [unwired: 2 in, 1 out]
  n361 = call "Initialize 1D Array (U64) from 1D Array (Variant).vi"() -> ()  [unwired: 2 in, 1 out]
  n362 = call "Initialize 1D Array (U64) from 1D Array (U8).vi"() -> ()  [unwired: 2 in, 1 out]
  n363 = call "Initialize 1D Array (U64) from 1D Array (U64).vi"() -> ()  [unwired: 2 in, 1 out]
  n364 = call "Initialize 1D Array (U64) from 1D Array (U32).vi"() -> ()  [unwired: 2 in, 1 out]
  n365 = call "Initialize 1D Array (U64) from 1D Array (U16).vi"() -> ()  [unwired: 2 in, 1 out]
  n366 = call "Initialize 1D Array (U64) from 1D Array (String).vi"() -> ()  [unwired: 2 in, 1 out]
  n367 = call "Initialize 1D Array (U64) from 1D Array (SGL).vi"() -> ()  [unwired: 2 in, 1 out]
  n368 = call "Initialize 1D Array (U64) from 1D Array (Path).vi"() -> ()  [unwired: 2 in, 1 out]
  n369 = call "Initialize 1D Array (U64) from 1D Array (I8).vi"() -> ()  [unwired: 2 in, 1 out]
  n370 = call "Initialize 1D Array (U64) from 1D Array (I64).vi"() -> ()  [unwired: 2 in, 1 out]
  n371 = call "Initialize 1D Array (U64) from 1D Array (I32).vi"() -> ()  [unwired: 2 in, 1 out]
  n372 = call "Initialize 1D Array (U64) from 1D Array (I16).vi"() -> ()  [unwired: 2 in, 1 out]
  n373 = call "Initialize 1D Array (U64) from 1D Array (EXT).vi"() -> ()  [unwired: 2 in, 1 out]
  n374 = call "Initialize 1D Array (U64) from 1D Array (DBL).vi"() -> ()  [unwired: 2 in, 1 out]
  n375 = call "Initialize 1D Array (U64) from 1D Array (CXT).vi"() -> ()  [unwired: 2 in, 1 out]
  n376 = call "Initialize 1D Array (U64) from 1D Array (CSG).vi"() -> ()  [unwired: 2 in, 1 out]
  n377 = call "Initialize 1D Array (U64) from 1D Array (CDB).vi"() -> ()  [unwired: 2 in, 1 out]
  n378 = call "Initialize 1D Array (U64) from 1D Array (Boolean).vi"() -> ()  [unwired: 2 in, 1 out]
  n379 = call "Initialize 1D Array (U32) from 1D Array (Variant).vi"() -> ()  [unwired: 2 in, 1 out]
  n380 = call "Initialize 1D Array (U32) from 1D Array (U8).vi"() -> ()  [unwired: 2 in, 1 out]
  n381 = call "Initialize 1D Array (U32) from 1D Array (U64).vi"() -> ()  [unwired: 2 in, 1 out]
  n382 = call "Initialize 1D Array (U32) from 1D Array (U32).vi"() -> ()  [unwired: 2 in, 1 out]
  n383 = call "Initialize 1D Array (U32) from 1D Array (U16).vi"() -> ()  [unwired: 2 in, 1 out]
  n384 = call "Initialize 1D Array (U32) from 1D Array (String).vi"() -> ()  [unwired: 2 in, 1 out]
  n385 = call "Initialize 1D Array (U32) from 1D Array (SGL).vi"() -> ()  [unwired: 2 in, 1 out]
  n386 = call "Initialize 1D Array (U32) from 1D Array (Path).vi"() -> ()  [unwired: 2 in, 1 out]
  n387 = call "Initialize 1D Array (U32) from 1D Array (I8).vi"() -> ()  [unwired: 2 in, 1 out]
  n388 = call "Initialize 1D Array (U32) from 1D Array (I64).vi"() -> ()  [unwired: 2 in, 1 out]
  n389 = call "Initialize 1D Array (U32) from 1D Array (I32).vi"() -> ()  [unwired: 2 in, 1 out]
  n390 = call "Initialize 1D Array (U32) from 1D Array (I16).vi"() -> ()  [unwired: 2 in, 1 out]
  n391 = call "Initialize 1D Array (U32) from 1D Array (EXT).vi"() -> ()  [unwired: 2 in, 1 out]
  n392 = call "Initialize 1D Array (U32) from 1D Array (DBL).vi"() -> ()  [unwired: 2 in, 1 out]
  n393 = call "Initialize 1D Array (U32) from 1D Array (CXT).vi"() -> ()  [unwired: 2 in, 1 out]
  n394 = call "Initialize 1D Array (U32) from 1D Array (CSG).vi"() -> ()  [unwired: 2 in, 1 out]
  n395 = call "Initialize 1D Array (U32) from 1D Array (CDB).vi"() -> ()  [unwired: 2 in, 1 out]
  n396 = call "Initialize 1D Array (U32) from 1D Array (Boolean).vi"() -> ()  [unwired: 2 in, 1 out]
  n397 = call "Initialize 1D Array (U16) from 1D Array (Variant).vi"() -> ()  [unwired: 2 in, 1 out]
  n398 = call "Initialize 1D Array (U16) from 1D Array (U8).vi"() -> ()  [unwired: 2 in, 1 out]
  n399 = call "Initialize 1D Array (U16) from 1D Array (U64).vi"() -> ()  [unwired: 2 in, 1 out]
  n400 = call "Initialize 1D Array (U16) from 1D Array (U32).vi"() -> ()  [unwired: 2 in, 1 out]
  n401 = call "Initialize 1D Array (U16) from 1D Array (U16).vi"() -> ()  [unwired: 2 in, 1 out]
  n402 = call "Initialize 1D Array (U16) from 1D Array (String).vi"() -> ()  [unwired: 2 in, 1 out]
  n403 = call "Initialize 1D Array (U16) from 1D Array (SGL).vi"() -> ()  [unwired: 2 in, 1 out]
  n404 = call "Initialize 1D Array (U16) from 1D Array (Path).vi"() -> ()  [unwired: 2 in, 1 out]
  n405 = call "Initialize 1D Array (U16) from 1D Array (I8).vi"() -> ()  [unwired: 2 in, 1 out]
  n406 = call "Initialize 1D Array (U16) from 1D Array (I64).vi"() -> ()  [unwired: 2 in, 1 out]
  n407 = call "Initialize 1D Array (U16) from 1D Array (I32).vi"() -> ()  [unwired: 2 in, 1 out]
  n408 = call "Initialize 1D Array (U16) from 1D Array (I16).vi"() -> ()  [unwired: 2 in, 1 out]
  n409 = call "Initialize 1D Array (U16) from 1D Array (EXT).vi"() -> ()  [unwired: 2 in, 1 out]
  n410 = call "Initialize 1D Array (U16) from 1D Array (DBL).vi"() -> ()  [unwired: 2 in, 1 out]
  n411 = call "Initialize 1D Array (U16) from 1D Array (CXT).vi"() -> ()  [unwired: 2 in, 1 out]
  n412 = call "Initialize 1D Array (U16) from 1D Array (CSG).vi"() -> ()  [unwired: 2 in, 1 out]
  n413 = call "Initialize 1D Array (U16) from 1D Array (CDB).vi"() -> ()  [unwired: 2 in, 1 out]
  n414 = call "Initialize 1D Array (U16) from 1D Array (Boolean).vi"() -> ()  [unwired: 2 in, 1 out]
  n415 = call "Initialize 1D Array (String) from 1D Array (Variant).vi"() -> ()  [unwired: 2 in, 1 out]
  n416 = call "Initialize 1D Array (String) from 1D Array (U8).vi"() -> ()  [unwired: 2 in, 1 out]
  n417 = call "Initialize 1D Array (String) from 1D Array (U64).vi"() -> ()  [unwired: 2 in, 1 out]
  n418 = call "Initialize 1D Array (String) from 1D Array (U32).vi"() -> ()  [unwired: 2 in, 1 out]
  n419 = call "Initialize 1D Array (String) from 1D Array (U16).vi"() -> ()  [unwired: 2 in, 1 out]
  n420 = call "Initialize 1D Array (String) from 1D Array (String).vi"() -> ()  [unwired: 2 in, 1 out]
  n421 = call "Initialize 1D Array (String) from 1D Array (SGL).vi"() -> ()  [unwired: 2 in, 1 out]
  n422 = call "Initialize 1D Array (String) from 1D Array (Path).vi"() -> ()  [unwired: 2 in, 1 out]
  n423 = call "Initialize 1D Array (String) from 1D Array (I8).vi"() -> ()  [unwired: 2 in, 1 out]
  n424 = call "Initialize 1D Array (String) from 1D Array (I64).vi"() -> ()  [unwired: 2 in, 1 out]
  n425 = call "Initialize 1D Array (String) from 1D Array (I32).vi"() -> ()  [unwired: 2 in, 1 out]
  n426 = call "Initialize 1D Array (String) from 1D Array (I16).vi"() -> ()  [unwired: 2 in, 1 out]
  n427 = call "Initialize 1D Array (String) from 1D Array (EXT).vi"() -> ()  [unwired: 2 in, 1 out]
  n428 = call "Initialize 1D Array (String) from 1D Array (DBL).vi"() -> ()  [unwired: 2 in, 1 out]
  n429 = call "Initialize 1D Array (String) from 1D Array (CXT).vi"() -> ()  [unwired: 2 in, 1 out]
  n430 = call "Initialize 1D Array (String) from 1D Array (CSG).vi"() -> ()  [unwired: 2 in, 1 out]
  n431 = call "Initialize 1D Array (String) from 1D Array (CDB).vi"() -> ()  [unwired: 2 in, 1 out]
  n432 = call "Initialize 1D Array (String) from 1D Array (Boolean).vi"() -> ()  [unwired: 2 in, 1 out]
  n433 = call "Initialize 1D Array (SGL) from 1D Array (Variant).vi"() -> ()  [unwired: 2 in, 1 out]
  n434 = call "Initialize 1D Array (SGL) from 1D Array (U8).vi"() -> ()  [unwired: 2 in, 1 out]
  n435 = call "Initialize 1D Array (SGL) from 1D Array (U64).vi"() -> ()  [unwired: 2 in, 1 out]
  n436 = call "Initialize 1D Array (SGL) from 1D Array (U32).vi"() -> ()  [unwired: 2 in, 1 out]
  n437 = call "Initialize 1D Array (SGL) from 1D Array (U16).vi"() -> ()  [unwired: 2 in, 1 out]
  n438 = call "Initialize 1D Array (SGL) from 1D Array (String).vi"() -> ()  [unwired: 2 in, 1 out]
  n439 = call "Initialize 1D Array (SGL) from 1D Array (SGL).vi"() -> ()  [unwired: 2 in, 1 out]
  n440 = call "Initialize 1D Array (SGL) from 1D Array (Path).vi"() -> ()  [unwired: 2 in, 1 out]
  n441 = call "Initialize 1D Array (SGL) from 1D Array (I8).vi"() -> ()  [unwired: 2 in, 1 out]
  n442 = call "Initialize 1D Array (SGL) from 1D Array (I64).vi"() -> ()  [unwired: 2 in, 1 out]
  n443 = call "Initialize 1D Array (SGL) from 1D Array (I32).vi"() -> ()  [unwired: 2 in, 1 out]
  n444 = call "Initialize 1D Array (SGL) from 1D Array (I16).vi"() -> ()  [unwired: 2 in, 1 out]
  n445 = call "Initialize 1D Array (SGL) from 1D Array (EXT).vi"() -> ()  [unwired: 2 in, 1 out]
  n446 = call "Initialize 1D Array (SGL) from 1D Array (DBL).vi"() -> ()  [unwired: 2 in, 1 out]
  n447 = call "Initialize 1D Array (SGL) from 1D Array (CXT).vi"() -> ()  [unwired: 2 in, 1 out]
  n448 = call "Initialize 1D Array (SGL) from 1D Array (CSG).vi"() -> ()  [unwired: 2 in, 1 out]
  n449 = call "Initialize 1D Array (SGL) from 1D Array (CDB).vi"() -> ()  [unwired: 2 in, 1 out]
  n450 = call "Initialize 1D Array (SGL) from 1D Array (Boolean).vi"() -> ()  [unwired: 2 in, 1 out]
  n451 = call "Initialize 1D Array (Path) from 1D Array (Variant).vi"() -> ()  [unwired: 2 in, 1 out]
  n452 = call "Initialize 1D Array (Path) from 1D Array (U8).vi"() -> ()  [unwired: 2 in, 1 out]
  n453 = call "Initialize 1D Array (Path) from 1D Array (U64).vi"() -> ()  [unwired: 2 in, 1 out]
  n454 = call "Initialize 1D Array (Path) from 1D Array (U32).vi"() -> ()  [unwired: 2 in, 1 out]
  n455 = call "Initialize 1D Array (Path) from 1D Array (U16).vi"() -> ()  [unwired: 2 in, 1 out]
  n456 = call "Initialize 1D Array (Path) from 1D Array (String).vi"() -> ()  [unwired: 2 in, 1 out]
  n457 = call "Initialize 1D Array (Path) from 1D Array (SGL).vi"() -> ()  [unwired: 2 in, 1 out]
  n458 = call "Initialize 1D Array (Path) from 1D Array (Path).vi"() -> ()  [unwired: 2 in, 1 out]
  n459 = call "Initialize 1D Array (Path) from 1D Array (I8).vi"() -> ()  [unwired: 2 in, 1 out]
  n460 = call "Initialize 1D Array (Path) from 1D Array (I64).vi"() -> ()  [unwired: 2 in, 1 out]
  n461 = call "Initialize 1D Array (Path) from 1D Array (I32).vi"() -> ()  [unwired: 2 in, 1 out]
  n462 = call "Initialize 1D Array (Path) from 1D Array (I16).vi"() -> ()  [unwired: 2 in, 1 out]
  n463 = call "Initialize 1D Array (Path) from 1D Array (EXT).vi"() -> ()  [unwired: 2 in, 1 out]
  n464 = call "Initialize 1D Array (Path) from 1D Array (DBL).vi"() -> ()  [unwired: 2 in, 1 out]
  n465 = call "Initialize 1D Array (Path) from 1D Array (CXT).vi"() -> ()  [unwired: 2 in, 1 out]
  n466 = call "Initialize 1D Array (Path) from 1D Array (CSG).vi"() -> ()  [unwired: 2 in, 1 out]
  n467 = call "Initialize 1D Array (Path) from 1D Array (CDB).vi"() -> ()  [unwired: 2 in, 1 out]
  n468 = call "Initialize 1D Array (Path) from 1D Array (Boolean).vi"() -> ()  [unwired: 2 in, 1 out]
  n469 = call "Initialize 1D Array (I8) from 1D Array (Variant).vi"() -> ()  [unwired: 2 in, 1 out]
  n470 = call "Initialize 1D Array (I8) from 1D Array (U8).vi"() -> ()  [unwired: 2 in, 1 out]
  n471 = call "Initialize 1D Array (I8) from 1D Array (U64).vi"() -> ()  [unwired: 2 in, 1 out]
  n472 = call "Initialize 1D Array (I8) from 1D Array (U32).vi"() -> ()  [unwired: 2 in, 1 out]
  n473 = call "Initialize 1D Array (I8) from 1D Array (U16).vi"() -> ()  [unwired: 2 in, 1 out]
  n474 = call "Initialize 1D Array (I8) from 1D Array (String).vi"() -> ()  [unwired: 2 in, 1 out]
  n475 = call "Initialize 1D Array (I8) from 1D Array (SGL).vi"() -> ()  [unwired: 2 in, 1 out]
  n476 = call "Initialize 1D Array (I8) from 1D Array (Path).vi"() -> ()  [unwired: 2 in, 1 out]
  n477 = call "Initialize 1D Array (I8) from 1D Array (I8).vi"() -> ()  [unwired: 2 in, 1 out]
  n478 = call "Initialize 1D Array (I8) from 1D Array (I64).vi"() -> ()  [unwired: 2 in, 1 out]
  n479 = call "Initialize 1D Array (I8) from 1D Array (I32).vi"() -> ()  [unwired: 2 in, 1 out]
  n480 = call "Initialize 1D Array (I8) from 1D Array (I16).vi"() -> ()  [unwired: 2 in, 1 out]
  n481 = call "Initialize 1D Array (I8) from 1D Array (EXT).vi"() -> ()  [unwired: 2 in, 1 out]
  n482 = call "Initialize 1D Array (I8) from 1D Array (DBL).vi"() -> ()  [unwired: 2 in, 1 out]
  n483 = call "Initialize 1D Array (I8) from 1D Array (CXT).vi"() -> ()  [unwired: 2 in, 1 out]
  n484 = call "Initialize 1D Array (I8) from 1D Array (CSG).vi"() -> ()  [unwired: 2 in, 1 out]
  n485 = call "Initialize 1D Array (I8) from 1D Array (CDB).vi"() -> ()  [unwired: 2 in, 1 out]
  n486 = call "Initialize 1D Array (I8) from 1D Array (Boolean).vi"() -> ()  [unwired: 2 in, 1 out]
  n487 = call "Initialize 1D Array (I64) from 1D Array (Variant).vi"() -> ()  [unwired: 2 in, 1 out]
  n488 = call "Initialize 1D Array (I64) from 1D Array (U8).vi"() -> ()  [unwired: 2 in, 1 out]
  n489 = call "Initialize 1D Array (I64) from 1D Array (U64).vi"() -> ()  [unwired: 2 in, 1 out]
  n490 = call "Initialize 1D Array (I64) from 1D Array (U32).vi"() -> ()  [unwired: 2 in, 1 out]
  n491 = call "Initialize 1D Array (I64) from 1D Array (U16).vi"() -> ()  [unwired: 2 in, 1 out]
  n492 = call "Initialize 1D Array (I64) from 1D Array (String).vi"() -> ()  [unwired: 2 in, 1 out]
  n493 = call "Initialize 1D Array (I64) from 1D Array (SGL).vi"() -> ()  [unwired: 2 in, 1 out]
  n494 = call "Initialize 1D Array (I64) from 1D Array (Path).vi"() -> ()  [unwired: 2 in, 1 out]
  n495 = call "Initialize 1D Array (I64) from 1D Array (I8).vi"() -> ()  [unwired: 2 in, 1 out]
  n496 = call "Initialize 1D Array (I64) from 1D Array (I64).vi"() -> ()  [unwired: 2 in, 1 out]
  n497 = call "Initialize 1D Array (I64) from 1D Array (I32).vi"() -> ()  [unwired: 2 in, 1 out]
  n498 = call "Initialize 1D Array (I64) from 1D Array (I16).vi"() -> ()  [unwired: 2 in, 1 out]
  n499 = call "Initialize 1D Array (I64) from 1D Array (EXT).vi"() -> ()  [unwired: 2 in, 1 out]
  n500 = call "Initialize 1D Array (I64) from 1D Array (DBL).vi"() -> ()  [unwired: 2 in, 1 out]
  n501 = call "Initialize 1D Array (I64) from 1D Array (CXT).vi"() -> ()  [unwired: 2 in, 1 out]
  n502 = call "Initialize 1D Array (I64) from 1D Array (CSG).vi"() -> ()  [unwired: 2 in, 1 out]
  n503 = call "Initialize 1D Array (I64) from 1D Array (CDB).vi"() -> ()  [unwired: 2 in, 1 out]
  n504 = call "Initialize 1D Array (I64) from 1D Array (Boolean).vi"() -> ()  [unwired: 2 in, 1 out]
  n505 = call "Initialize 1D Array (I32) from 1D Array (Variant).vi"() -> ()  [unwired: 2 in, 1 out]
  n506 = call "Initialize 1D Array (I32) from 1D Array (U8).vi"() -> ()  [unwired: 2 in, 1 out]
  n507 = call "Initialize 1D Array (I32) from 1D Array (U64).vi"() -> ()  [unwired: 2 in, 1 out]
  n508 = call "Initialize 1D Array (I32) from 1D Array (U32).vi"() -> ()  [unwired: 2 in, 1 out]
  n509 = call "Initialize 1D Array (I32) from 1D Array (U16).vi"() -> ()  [unwired: 2 in, 1 out]
  n510 = call "Initialize 1D Array (I32) from 1D Array (String).vi"() -> ()  [unwired: 2 in, 1 out]
  n511 = call "Initialize 1D Array (I32) from 1D Array (SGL).vi"() -> ()  [unwired: 2 in, 1 out]
  n512 = call "Initialize 1D Array (I32) from 1D Array (Path).vi"() -> ()  [unwired: 2 in, 1 out]
  n513 = call "Initialize 1D Array (I32) from 1D Array (I8).vi"() -> ()  [unwired: 2 in, 1 out]
  n514 = call "Initialize 1D Array (I32) from 1D Array (I64).vi"() -> ()  [unwired: 2 in, 1 out]
  n515 = call "Initialize 1D Array (I32) from 1D Array (I32).vi"() -> ()  [unwired: 2 in, 1 out]
  n516 = call "Initialize 1D Array (I32) from 1D Array (I16).vi"() -> ()  [unwired: 2 in, 1 out]
  n517 = call "Initialize 1D Array (I32) from 1D Array (EXT).vi"() -> ()  [unwired: 2 in, 1 out]
  n518 = call "Initialize 1D Array (I32) from 1D Array (DBL).vi"() -> ()  [unwired: 2 in, 1 out]
  n519 = call "Initialize 1D Array (I32) from 1D Array (CXT).vi"() -> ()  [unwired: 2 in, 1 out]
  n520 = call "Initialize 1D Array (I32) from 1D Array (CSG).vi"() -> ()  [unwired: 2 in, 1 out]
  n521 = call "Initialize 1D Array (I32) from 1D Array (CDB).vi"() -> ()  [unwired: 2 in, 1 out]
  n522 = call "Initialize 1D Array (I32) from 1D Array (Boolean).vi"() -> ()  [unwired: 2 in, 1 out]
  n523 = call "Initialize 1D Array (I16) from 1D Array (Variant).vi"() -> ()  [unwired: 2 in, 1 out]
  n524 = call "Initialize 1D Array (I16) from 1D Array (U8).vi"() -> ()  [unwired: 2 in, 1 out]
  n525 = call "Initialize 1D Array (I16) from 1D Array (U64).vi"() -> ()  [unwired: 2 in, 1 out]
  n526 = call "Initialize 1D Array (I16) from 1D Array (U32).vi"() -> ()  [unwired: 2 in, 1 out]
  n527 = call "Initialize 1D Array (I16) from 1D Array (U16).vi"() -> ()  [unwired: 2 in, 1 out]
  n528 = call "Initialize 1D Array (I16) from 1D Array (String).vi"() -> ()  [unwired: 2 in, 1 out]
  n529 = call "Initialize 1D Array (I16) from 1D Array (SGL).vi"() -> ()  [unwired: 2 in, 1 out]
  n530 = call "Initialize 1D Array (I16) from 1D Array (Path).vi"() -> ()  [unwired: 2 in, 1 out]
  n531 = call "Initialize 1D Array (I16) from 1D Array (I8).vi"() -> ()  [unwired: 2 in, 1 out]
  n532 = call "Initialize 1D Array (I16) from 1D Array (I64).vi"() -> ()  [unwired: 2 in, 1 out]
  n533 = call "Initialize 1D Array (I16) from 1D Array (I32).vi"() -> ()  [unwired: 2 in, 1 out]
  n534 = call "Initialize 1D Array (I16) from 1D Array (I16).vi"() -> ()  [unwired: 2 in, 1 out]
  n535 = call "Initialize 1D Array (I16) from 1D Array (EXT).vi"() -> ()  [unwired: 2 in, 1 out]
  n536 = call "Initialize 1D Array (I16) from 1D Array (DBL).vi"() -> ()  [unwired: 2 in, 1 out]
  n537 = call "Initialize 1D Array (I16) from 1D Array (CXT).vi"() -> ()  [unwired: 2 in, 1 out]
  n538 = call "Initialize 1D Array (I16) from 1D Array (CSG).vi"() -> ()  [unwired: 2 in, 1 out]
  n539 = call "Initialize 1D Array (I16) from 1D Array (CDB).vi"() -> ()  [unwired: 2 in, 1 out]
  n540 = call "Initialize 1D Array (I16) from 1D Array (Boolean).vi"() -> ()  [unwired: 2 in, 1 out]
  n541 = call "Initialize 1D Array (EXT) from 1D Array (Variant).vi"() -> ()  [unwired: 2 in, 1 out]
  n542 = call "Initialize 1D Array (EXT) from 1D Array (U8).vi"() -> ()  [unwired: 2 in, 1 out]
  n543 = call "Initialize 1D Array (EXT) from 1D Array (U64).vi"() -> ()  [unwired: 2 in, 1 out]
  n544 = call "Initialize 1D Array (EXT) from 1D Array (U32).vi"() -> ()  [unwired: 2 in, 1 out]
  n545 = call "Initialize 1D Array (EXT) from 1D Array (U16).vi"() -> ()  [unwired: 2 in, 1 out]
  n546 = call "Initialize 1D Array (EXT) from 1D Array (String).vi"() -> ()  [unwired: 2 in, 1 out]
  n547 = call "Initialize 1D Array (EXT) from 1D Array (SGL).vi"() -> ()  [unwired: 2 in, 1 out]
  n548 = call "Initialize 1D Array (EXT) from 1D Array (Path).vi"() -> ()  [unwired: 2 in, 1 out]
  n549 = call "Initialize 1D Array (EXT) from 1D Array (I8).vi"() -> ()  [unwired: 2 in, 1 out]
  n550 = call "Initialize 1D Array (EXT) from 1D Array (I64).vi"() -> ()  [unwired: 2 in, 1 out]
  n551 = call "Initialize 1D Array (EXT) from 1D Array (I32).vi"() -> ()  [unwired: 2 in, 1 out]
  n552 = call "Initialize 1D Array (EXT) from 1D Array (I16).vi"() -> ()  [unwired: 2 in, 1 out]
  n553 = call "Initialize 1D Array (EXT) from 1D Array (EXT).vi"() -> ()  [unwired: 2 in, 1 out]
  n554 = call "Initialize 1D Array (EXT) from 1D Array (DBL).vi"() -> ()  [unwired: 2 in, 1 out]
  n555 = call "Initialize 1D Array (EXT) from 1D Array (CXT).vi"() -> ()  [unwired: 2 in, 1 out]
  n556 = call "Initialize 1D Array (EXT) from 1D Array (CSG).vi"() -> ()  [unwired: 2 in, 1 out]
  n557 = call "Initialize 1D Array (EXT) from 1D Array (CDB).vi"() -> ()  [unwired: 2 in, 1 out]
  n558 = call "Initialize 1D Array (EXT) from 1D Array (Boolean).vi"() -> ()  [unwired: 2 in, 1 out]
  n559 = call "Initialize 1D Array (DBL) from 1D Array (Variant).vi"() -> ()  [unwired: 2 in, 1 out]
  n560 = call "Initialize 1D Array (DBL) from 1D Array (U8).vi"() -> ()  [unwired: 2 in, 1 out]
  n561 = call "Initialize 1D Array (DBL) from 1D Array (U64).vi"() -> ()  [unwired: 2 in, 1 out]
  n562 = call "Initialize 1D Array (DBL) from 1D Array (U32).vi"() -> ()  [unwired: 2 in, 1 out]
  n563 = call "Initialize 1D Array (DBL) from 1D Array (U16).vi"() -> ()  [unwired: 2 in, 1 out]
  n564 = call "Initialize 1D Array (DBL) from 1D Array (String).vi"() -> ()  [unwired: 2 in, 1 out]
  n565 = call "Initialize 1D Array (DBL) from 1D Array (SGL).vi"() -> ()  [unwired: 2 in, 1 out]
  n566 = call "Initialize 1D Array (DBL) from 1D Array (Path).vi"() -> ()  [unwired: 2 in, 1 out]
  n567 = call "Initialize 1D Array (DBL) from 1D Array (I8).vi"() -> ()  [unwired: 2 in, 1 out]
  n568 = call "Initialize 1D Array (DBL) from 1D Array (I64).vi"() -> ()  [unwired: 2 in, 1 out]
  n569 = call "Initialize 1D Array (DBL) from 1D Array (I32).vi"() -> ()  [unwired: 2 in, 1 out]
  n570 = call "Initialize 1D Array (DBL) from 1D Array (I16).vi"() -> ()  [unwired: 2 in, 1 out]
  n571 = call "Initialize 1D Array (DBL) from 1D Array (EXT).vi"() -> ()  [unwired: 2 in, 1 out]
  n572 = call "Initialize 1D Array (DBL) from 1D Array (DBL).vi"() -> ()  [unwired: 2 in, 1 out]
  n573 = call "Initialize 1D Array (DBL) from 1D Array (CXT).vi"() -> ()  [unwired: 2 in, 1 out]
  n574 = call "Initialize 1D Array (DBL) from 1D Array (CSG).vi"() -> ()  [unwired: 2 in, 1 out]
  n575 = call "Initialize 1D Array (DBL) from 1D Array (CDB).vi"() -> ()  [unwired: 2 in, 1 out]
  n576 = call "Initialize 1D Array (DBL) from 1D Array (Boolean).vi"() -> ()  [unwired: 2 in, 1 out]
  n577 = call "Initialize 1D Array (CXT) from 1D Array (Variant).vi"() -> ()  [unwired: 2 in, 1 out]
  n578 = call "Initialize 1D Array (CXT) from 1D Array (U8).vi"() -> ()  [unwired: 2 in, 1 out]
  n579 = call "Initialize 1D Array (CXT) from 1D Array (U64).vi"() -> ()  [unwired: 2 in, 1 out]
  n580 = call "Initialize 1D Array (CXT) from 1D Array (U32).vi"() -> ()  [unwired: 2 in, 1 out]
  n581 = call "Initialize 1D Array (CXT) from 1D Array (U16).vi"() -> ()  [unwired: 2 in, 1 out]
  n582 = call "Initialize 1D Array (CXT) from 1D Array (String).vi"() -> ()  [unwired: 2 in, 1 out]
  n583 = call "Initialize 1D Array (CXT) from 1D Array (SGL).vi"() -> ()  [unwired: 2 in, 1 out]
  n584 = call "Initialize 1D Array (CXT) from 1D Array (Path).vi"() -> ()  [unwired: 2 in, 1 out]
  n585 = call "Initialize 1D Array (CXT) from 1D Array (I8).vi"() -> ()  [unwired: 2 in, 1 out]
  n586 = call "Initialize 1D Array (CXT) from 1D Array (I64).vi"() -> ()  [unwired: 2 in, 1 out]
  n587 = call "Initialize 1D Array (CXT) from 1D Array (I32).vi"() -> ()  [unwired: 2 in, 1 out]
  n588 = call "Initialize 1D Array (CXT) from 1D Array (I16).vi"() -> ()  [unwired: 2 in, 1 out]
  n589 = call "Initialize 1D Array (CXT) from 1D Array (EXT).vi"() -> ()  [unwired: 2 in, 1 out]
  n590 = call "Initialize 1D Array (CXT) from 1D Array (DBL).vi"() -> ()  [unwired: 2 in, 1 out]
  n591 = call "Initialize 1D Array (CXT) from 1D Array (CXT).vi"() -> ()  [unwired: 2 in, 1 out]
  n592 = call "Initialize 1D Array (CXT) from 1D Array (CSG).vi"() -> ()  [unwired: 2 in, 1 out]
  n593 = call "Initialize 1D Array (CXT) from 1D Array (CDB).vi"() -> ()  [unwired: 2 in, 1 out]
  n594 = call "Initialize 1D Array (CXT) from 1D Array (Boolean).vi"() -> ()  [unwired: 2 in, 1 out]
  n595 = call "Initialize 1D Array (CSG) from 1D Array (Variant).vi"() -> ()  [unwired: 2 in, 1 out]
  n596 = call "Initialize 1D Array (CSG) from 1D Array (U8).vi"() -> ()  [unwired: 2 in, 1 out]
  n597 = call "Initialize 1D Array (CSG) from 1D Array (U64).vi"() -> ()  [unwired: 2 in, 1 out]
  n598 = call "Initialize 1D Array (CSG) from 1D Array (U32).vi"() -> ()  [unwired: 2 in, 1 out]
  n599 = call "Initialize 1D Array (CSG) from 1D Array (U16).vi"() -> ()  [unwired: 2 in, 1 out]
  n600 = call "Initialize 1D Array (CSG) from 1D Array (String).vi"() -> ()  [unwired: 2 in, 1 out]
  n601 = call "Initialize 1D Array (CSG) from 1D Array (SGL).vi"() -> ()  [unwired: 2 in, 1 out]
  n602 = call "Initialize 1D Array (CSG) from 1D Array (Path).vi"() -> ()  [unwired: 2 in, 1 out]
  n603 = call "Initialize 1D Array (CSG) from 1D Array (I8).vi"() -> ()  [unwired: 2 in, 1 out]
  n604 = call "Initialize 1D Array (CSG) from 1D Array (I64).vi"() -> ()  [unwired: 2 in, 1 out]
  n605 = call "Initialize 1D Array (CSG) from 1D Array (I32).vi"() -> ()  [unwired: 2 in, 1 out]
  n606 = call "Initialize 1D Array (CSG) from 1D Array (I16).vi"() -> ()  [unwired: 2 in, 1 out]
  n607 = call "Initialize 1D Array (CSG) from 1D Array (EXT).vi"() -> ()  [unwired: 2 in, 1 out]
  n608 = call "Initialize 1D Array (CSG) from 1D Array (DBL).vi"() -> ()  [unwired: 2 in, 1 out]
  n609 = call "Initialize 1D Array (CSG) from 1D Array (CXT).vi"() -> ()  [unwired: 2 in, 1 out]
  n610 = call "Initialize 1D Array (CSG) from 1D Array (CSG).vi"() -> ()  [unwired: 2 in, 1 out]
  n611 = call "Initialize 1D Array (CSG) from 1D Array (CDB).vi"() -> ()  [unwired: 2 in, 1 out]
  n612 = call "Initialize 1D Array (CSG) from 1D Array (Boolean).vi"() -> ()  [unwired: 2 in, 1 out]
  n613 = call "Initialize 1D Array (CDB) from 1D Array (Variant).vi"() -> ()  [unwired: 2 in, 1 out]
  n614 = call "Initialize 1D Array (CDB) from 1D Array (U8).vi"() -> ()  [unwired: 2 in, 1 out]
  n615 = call "Initialize 1D Array (CDB) from 1D Array (U64).vi"() -> ()  [unwired: 2 in, 1 out]
  n616 = call "Initialize 1D Array (CDB) from 1D Array (U32).vi"() -> ()  [unwired: 2 in, 1 out]
  n617 = call "Initialize 1D Array (CDB) from 1D Array (U16).vi"() -> ()  [unwired: 2 in, 1 out]
  n618 = call "Initialize 1D Array (CDB) from 1D Array (String).vi"() -> ()  [unwired: 2 in, 1 out]
  n619 = call "Initialize 1D Array (CDB) from 1D Array (SGL).vi"() -> ()  [unwired: 2 in, 1 out]
  n620 = call "Initialize 1D Array (CDB) from 1D Array (Path).vi"() -> ()  [unwired: 2 in, 1 out]
  n621 = call "Initialize 1D Array (CDB) from 1D Array (I8).vi"() -> ()  [unwired: 2 in, 1 out]
  n622 = call "Initialize 1D Array (CDB) from 1D Array (I64).vi"() -> ()  [unwired: 2 in, 1 out]
  n623 = call "Initialize 1D Array (CDB) from 1D Array (I32).vi"() -> ()  [unwired: 2 in, 1 out]
  n624 = call "Initialize 1D Array (CDB) from 1D Array (I16).vi"() -> ()  [unwired: 2 in, 1 out]
  n625 = call "Initialize 1D Array (CDB) from 1D Array (EXT).vi"() -> ()  [unwired: 2 in, 1 out]
  n626 = call "Initialize 1D Array (CDB) from 1D Array (DBL).vi"() -> ()  [unwired: 2 in, 1 out]
  n627 = call "Initialize 1D Array (CDB) from 1D Array (CXT).vi"() -> ()  [unwired: 2 in, 1 out]
  n628 = call "Initialize 1D Array (CDB) from 1D Array (CSG).vi"() -> ()  [unwired: 2 in, 1 out]
  n629 = call "Initialize 1D Array (CDB) from 1D Array (CDB).vi"() -> ()  [unwired: 2 in, 1 out]
  n630 = call "Initialize 1D Array (CDB) from 1D Array (Boolean).vi"() -> ()  [unwired: 2 in, 1 out]
  n631 = call "Initialize 1D Array (Boolean) from 1D Array (Variant).vi"() -> ()  [unwired: 2 in, 1 out]
  n632 = call "Initialize 1D Array (Boolean) from 1D Array (U8).vi"() -> ()  [unwired: 2 in, 1 out]
  n633 = call "Initialize 1D Array (Boolean) from 1D Array (U64).vi"() -> ()  [unwired: 2 in, 1 out]
  n634 = call "Initialize 1D Array (Boolean) from 1D Array (U32).vi"() -> ()  [unwired: 2 in, 1 out]
  n635 = call "Initialize 1D Array (Boolean) from 1D Array (U16).vi"() -> ()  [unwired: 2 in, 1 out]
  n636 = call "Initialize 1D Array (Boolean) from 1D Array (String).vi"() -> ()  [unwired: 2 in, 1 out]
  n637 = call "Initialize 1D Array (Boolean) from 1D Array (SGL).vi"() -> ()  [unwired: 2 in, 1 out]
  n638 = call "Initialize 1D Array (Boolean) from 1D Array (Path).vi"() -> ()  [unwired: 2 in, 1 out]
  n639 = call "Initialize 1D Array (Boolean) from 1D Array (I8).vi"() -> ()  [unwired: 2 in, 1 out]
  n640 = call "Initialize 1D Array (Boolean) from 1D Array (I64).vi"() -> ()  [unwired: 2 in, 1 out]
  n641 = call "Initialize 1D Array (Boolean) from 1D Array (I32).vi"() -> ()  [unwired: 2 in, 1 out]
  n642 = call "Initialize 1D Array (Boolean) from 1D Array (I16).vi"() -> ()  [unwired: 2 in, 1 out]
  n643 = call "Initialize 1D Array (Boolean) from 1D Array (EXT).vi"() -> ()  [unwired: 2 in, 1 out]
  n644 = call "Initialize 1D Array (Boolean) from 1D Array (DBL).vi"() -> ()  [unwired: 2 in, 1 out]
  n645 = call "Initialize 1D Array (Boolean) from 1D Array (CXT).vi"() -> ()  [unwired: 2 in, 1 out]
  n646 = call "Initialize 1D Array (Boolean) from 1D Array (CSG).vi"() -> ()  [unwired: 2 in, 1 out]
  n647 = call "Initialize 1D Array (Boolean) from 1D Array (CDB).vi"() -> ()  [unwired: 2 in, 1 out]
  n648 = call "Initialize 1D Array (Boolean) from 1D Array (Boolean).vi"() -> ()  [unwired: 2 in, 1 out]
